vi "DAQ_shutter_write.vi"(3 "Error In":errorcluster, 4 "Collection Settings":T1, 5 "DAQmx Task Name":refnum<k21>) -> (0 "Error Out":errorcluster)   [LabVIEW 2018]
uses:
  Type defs/FileAcq_v1_Ctrl.ctl
  <vilib>/DAQmx/write.llb/DAQmx Write (Digital 1D Bool NChan 1Samp 1Line).vi
  <vilib>/DAQmx/miscellaneous.llb/DAQmx Fill In Error Info.vi
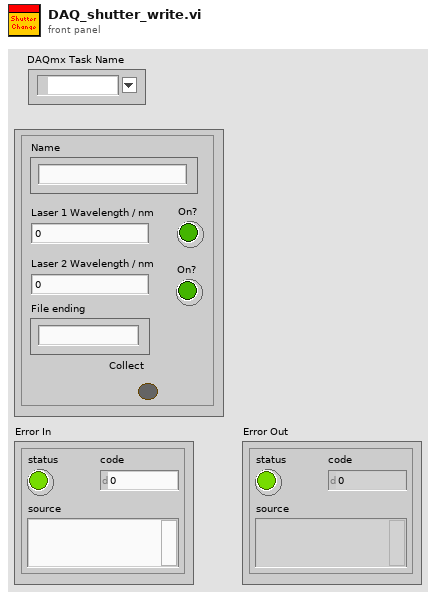
[diagram p1: front panel]
types:
  T1 = typedef "FileAcq_v1_Ctrl.ctl" = cluster{"Type":string, "LaserWave1":dbl, "Shutter1":bool, "LaserWave2":dbl, "Shutter2":bool, "FileEnd":string, "Collect":bool}
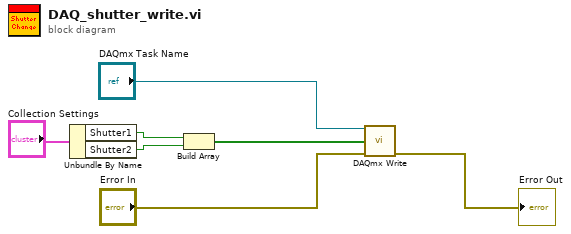
[diagram p0: block diagram]
diagram:
  n1 = Unbundle By Name("Collection Settings") -> ("Shutter1"=w6:bool, "Shutter2"=w5:bool)
  n2 = Build Array(w6, w5) -> (w4:bool[])
  n3 = call-poly <vilib>:"DAQmx Write.vi"("task/channels in"="DAQmx Task Name", "data"=w4, "error in"="Error In") -> ("error out"=→"Error Out":errorcluster)  [unwired: 10 in, 2 out]
